vi "Write L2 Enet FIFO.vi"(6 "FIFO Timestamps":T1, 8 "error in (no error)":errorcluster, 9 "Timeout (ms)":i32=100, 10 "Data in":u8[](array[numeric]), 11 "CIF_Fifo_L2Enet_Multi in":refnum<class "CIF_Fifo_L2Enet_Multi.lvclass">) -> (0 "error out":errorcluster, 1 "timed out?":bool, 3 "CIF_Fifo_L2Enet_Multi out":refnum<class "CIF_Fifo_L2Enet_Multi.lvclass">)   [LabVIEW 2021, in "CIF_Fifo_L2Enet_Multi.lvclass"]
uses:
  CIF_Fifo_L2Enet_Multi.lvclass
  D:/dev/Packages/Channel_Manager/src/CIFChannels/CIFChannels.lvclass
  ChannelCommon/typedef/TimeStamps.ctl
  CIF_Fifo_L2Enet_Multi.lvclass/CIF_Fifo_L2Enet_Multi.ctl
  CIFChannels/CIFChannels.lvclass/CIFChannels.ctl
  NIChn/CIF_NIChn.lvclass/CIF_NIChn.ctl
  <vilib>/CIF Foundation/CIF Utilities/Statistics/I64/Stats_I64_CIF_U.lvclass/Stats_I64_CIF_U.ctl
  369b2d9f-cd2a-4ce2-92c3-19653a73c8ad.vi
  e6281684-375c-44a7-85bc-c0cc59c3c0f1.vi
  ChannelCommon/Utilities/Unflatten Header.vi
  ChannelCommon/Utilities/Flatten Header.vi
  CIFChannels/Utilities/Update FIFO Header.vi
  NIChn/Accessors/Read CIF Channel.vi
  FIFO_U8/SubVIs/Core Write U8 FIFO.vi/1bad10da-a98b-49ee-b03a-18b497e396df.vi
  FIFO_U8/SubVIs/Core Write U8 FIFO.vi/70f860b1-5d4a-43dc-b0c2-c9446e8447f7.vi
  <vilib>/CIF Foundation/CIF Channels/CIFChannels/Top Level/Write U8 Array.vi
  CIFChannels/Accessors/Read FIFO Header.vi
  <vilib>/CIF Foundation/CIF Utilities/Statistics/I64/X1 minus X0.vi
  <vilib>/CIF Foundation/CIF Utilities/Time/System Time/Get System Time.vi
  <vilib>/CIF Foundation/CIF Utilities/DataTypes/Unflatten U64.vi
  <vilib>/CIF Foundation/CIF Utilities/DataTypes/Unflatten I64.vi
  ChannelCommon/Utilities/Add Error.vi
  <vilib>/CIF Foundation/CIF Utilities/DataTypes/Flatten U64.vi
  <vilib>/CIF Foundation/CIF Utilities/DataTypes/Flatten I64.vi
  <vilib>/CIF Foundation/CIF Channels/CIFChannels/SubVIs/Get dll Path.vi
  <vilib>/CIF Foundation/CIF Channels/CIFChannels/SubVIs/Get Requested Size.vi
  <vilib>/CIF Foundation/CIF Utilities/Statistics/I64/X1 minus X0.vi/dfabcf33-0dbc-4041-80a5-3dc0c86d2989.vi
  <vilib>/CIF Foundation/CIF Utilities/Time/System Time/LabVIEW Time to TAI Time.vi
  <vilib>/CIF Foundation/CIF Utilities/Errors/Append Error Location.vi
  <vilib>/CIF Foundation/CIF Utilities/Statistics/I64/X1 minus X0.vi/dfabcf33-0dbc-4041-80a5-3dc0c86d2989.vi/9eb60a9a-770f-4d2d-8b3f-8465c267ecc9.vi
  FIFO_U8/CIF_NIChn_Fifo_U8.lvclass
  D:/dev/Packages/Channel_Manager/src/CIF_NIChn/NIChn/CIF_NIChn.lvclass
  CIFChannels/CIFChannels.lvclass
  ChannelCommon/ChannelCommon.lvlib
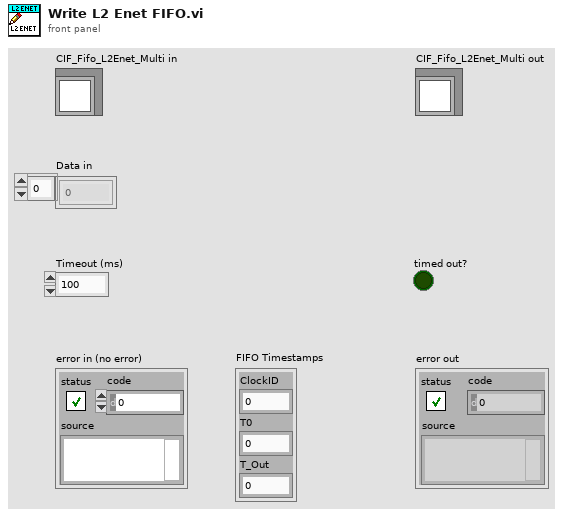
[diagram p1: front panel]
types:
  T1 = typedef "ChannelCommon.lvlib/TimeStamps.ctl" = cluster{"ClockID":u8, "T0":i64, "T_Out":i64}
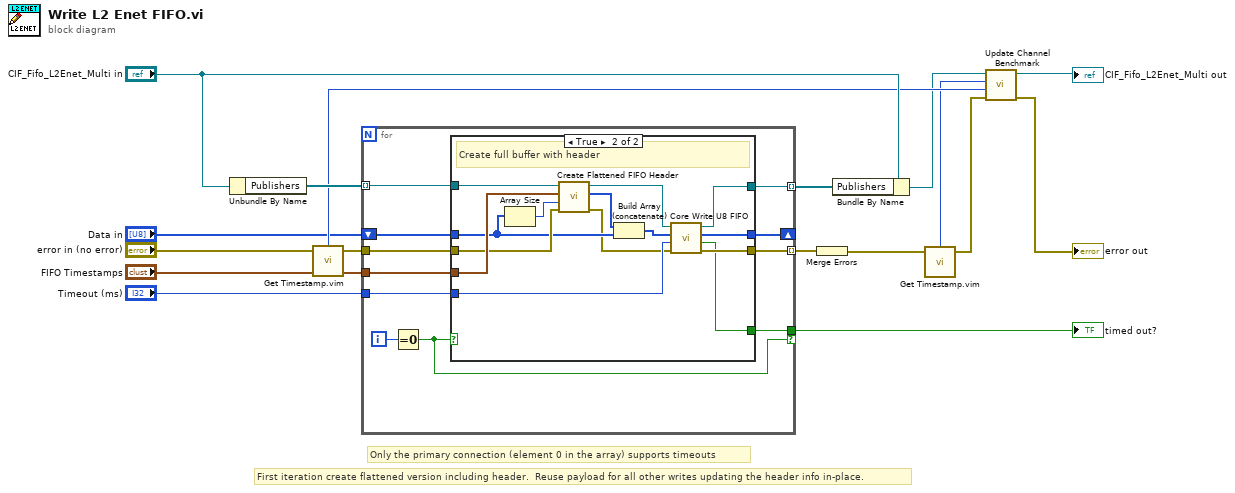
[diagram p0: block diagram]
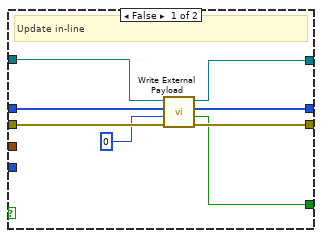
[diagram p2: hidden frame]
diagram:
  # "Only the primary connection (element 0 in the array) supports timeouts"
  # "First iteration create flattened version including header.  Reuse payload for all other writes updating the header info in-place."
  n1 = Unbundle By Name("CIF_Fifo_L2Enet_Multi in") -> ("Publishers"=w17:refnum<class "CIF_NIChn_Fifo_U8.lvclass">[])
  n2 = call "Get Timestamp.vim"("Anything in"="error in (no error)") -> ("Time (ns)"=w10:i64, "Anything out"=w6:errorcluster)  [unwired: 2 in]
  n3 = for {
    tunnel: w17 -> [w28] mode=indexing
    tunnel: [w26] -> w15 mode=indexing
    tunnel: [w25] -> w14 mode=indexing
    tunnel: w6 -> [w24]
    tunnel: "FIFO Timestamps" -> [w23]
    tunnel: "Timeout (ms)" -> [w21]
    tunnel: [w20] -> w11 if=w19
    shift-right: [w18] -> _
    shift-left: "Data in" -> [w27]
    i -> [w22]
    n4 = Equal To 0?(x=w22) -> (x = 0?=w19:bool)
    n5 = case shown="True" w19 {
      tunnel: w28 -> [w35 w50]
      tunnel: w27 -> [w32 w40]
      tunnel: [w34 w47] -> w26
      tunnel: [w33 w46] -> w25
      tunnel: w24 -> [w36 w42]
      tunnel: w23 -> [_ w49]
      tunnel: w21 -> [_ w44]
      tunnel: [w31 w45] -> w20
      tunnel: [w29 w37] -> w18
      frame False {
        # "Update in-line"
        n6 = call "Write External Payload.vi"("error in (no error)"=w36, "Timeout (ms)"=0, "U8 With Header in"=w32, "CIFFIFO in"=w35) -> ("error out"=w33:errorcluster, "timed out?"=w31:bool, "U8 With Header out"=w29:u8[], "CIFFIFO out"=w34:refnum<class "CIF_NIChn_Fifo_U8.lvclass">)  [unwired: 4 in]
      }
      frame True {
        # "Create full buffer with header"
        n7 = Array Size(array=w40) -> (size(s)=w43:i32)
        n8 = call "Create Flattened FIFO Header.vi"("error in (no error)"=w42, "Data Length"=w43, "FIFO Timestamps"=w49, "CIFChannels in"=w50) -> ("error out"=w39:errorcluster, "Flattened FIFO Header"=w41:u8[], "CIFChannels out"=w48:refnum<class "CIF_NIChn_Fifo_U8.lvclass">)  [unwired: 5 in]
        n9 = Build Array (concatenate)(w41, w40) -> (w38:u8[])
        n10 = call "Core Write U8 FIFO.vi"("error in (no error)"=w39, "Timeout (ms)"=w44, "U8 With Header in"=w38, "CIFFIFO in"=w48) -> ("error out"=w46:errorcluster, "timed out?"=w45:bool, "U8 With Header out"=w37:u8[], "CIFFIFO out"=w47:refnum<class "CIF_NIChn_Fifo_U8.lvclass">)  [unwired: 4 in]
      }
    }
  }
  "timed out?" <- w11
  n11 = Merge Errors(w14) -> (w5:errorcluster)
  n12 = Bundle By Name(cluster="CIF_Fifo_L2Enet_Multi in", "Publishers"=w15) -> (w3:refnum<class "CIF_Fifo_L2Enet_Multi.lvclass">)
  n13 = call "Get Timestamp.vim"("Anything in"=w5) -> ("Time (ns)"=w9:i64, "Anything out"=w8:errorcluster)  [unwired: 2 in]
  n14 = call "Update Channel Benchmark.vi"("error in (no error)"=w8, "X0"=w10, "X1"=w9, "CIFChannels in"=w3) -> ("error out"=→"error out":errorcluster, "CIFChannels out"=→"CIF_Fifo_L2Enet_Multi out":refnum<class "CIF_Fifo_L2Enet_Multi.lvclass">)  [unwired: 6 in]
